vi "GetHiSpeedDeviceGPIOs.vi"(0 "Handle":u32, 1 "error in (no error)":errorcluster) -> (2 "Result":u32, 3 "High IO Values":T1, 4 "error out":errorcluster)   [LabVIEW 2010]
uses:
  FTCSPI.dll
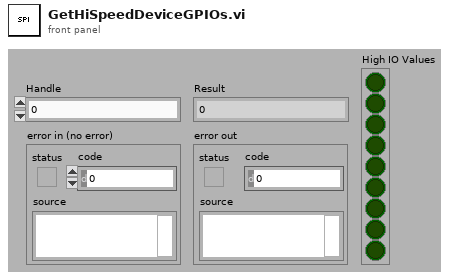
[diagram p1: front panel]
types:
  T1 = cluster{"[0]":bool, "[1]":bool, "[2]":bool, "[3]":bool, "[4]":bool, "[5]":bool, "[6]":bool, "[7]":bool, "[8]":bool}
  T2 = cluster{"Boolean":bool, "Boolean 2":bool, "Boolean 3":bool, "Boolean 4":bool, "Boolean 5":bool, "Boolean 6":bool, "Boolean 7":bool, "Boolean 8":bool}
  T3 = cluster{"[0]":u32, "[1]":u32, "[2]":u32, "[3]":u32, "[4]":u32, "[5]":u32, "[6]":u32, "[7]":u32, "[8]":u32}
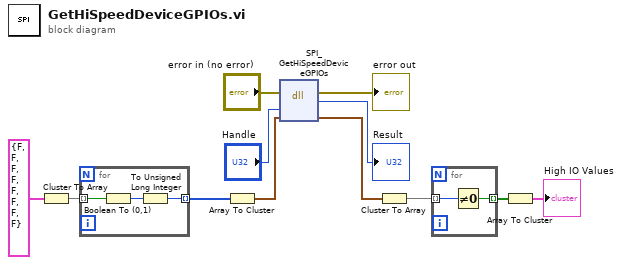
[diagram p0: block diagram]
diagram:
  n1 = Cluster To Array(cluster=T2 {"Boolean"=FALSE, "Boolean 2"=FALSE, "Boolean 3"=FALSE, "Boolean 4"=FALSE, "Boolean 5"=FALSE, "Boolean 6"=FALSE, "Boolean 7"=FALSE, "Boolean 8"=FALSE} ("High IO Values 2")) -> (array=w11:bool[])
  n2 = for {
    tunnel: w11 -> [w14] mode=indexing
    tunnel: [w13] -> w10 mode=indexing
    n3 = Boolean To (0,1)(Boolean=w14) -> (0, 1=w15:i16)
    n4 = To Unsigned Long Integer(number=w15) -> (unsigned 32bit integer=w13:u32)
  }
  n5 = Array To Cluster(array=w10) -> (cluster=w9:T3)
  n6 = dll-call lib="C:/Users/Administrator/Documents/GitHub/labview/FPGA/FTCSPI.dll" fn="SPI_GetHiSpeedDeviceGPIOs" label="SPI_GetGPIOs"(error in="error in (no error)", "handle"="Handle", "High Pins Data"=w9) -> (error out=→"error out":errorcluster, "result"=→"Result":u32, "High Pins Data"=w4:T3)  [unwired: 3 in, 1 out]
  n7 = Cluster To Array(cluster=w4) -> (array=w3:u32[])
  n8 = for {
    tunnel: w3 -> [w17] mode=indexing
    tunnel: [w16] -> w2 mode=indexing
    n9 = Not Equal To 0?(x=w17) -> (x != 0?=w16:bool)
  }
  n10 = Array To Cluster(array=w2) -> (cluster=→"High IO Values":T1)
